vi "Allocate Image Memory.vi"(11 "Reference Image File":string) -> (0 "error out":errorcluster, 1 "Reference Image":T1, 2 "HSL Threshold":T1, 3 "Acquisition Memory":T1[](array[typedef]), 5 "Mask":T1)   [LabVIEW 2018]
uses:
  <vilib>/vision/Image Controls.llb/IMAQ Image.ctl
panel:
  out "appended path":path
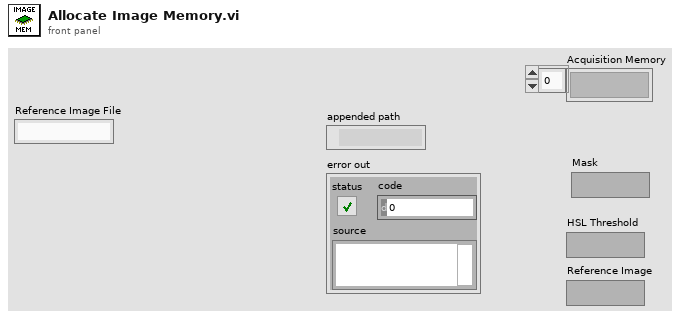
[diagram p1: front panel]
types:
  T1 = typedef "IMAQ Image.ctl" = refnum<image>
  T2 = typedef "Image Type" = u32
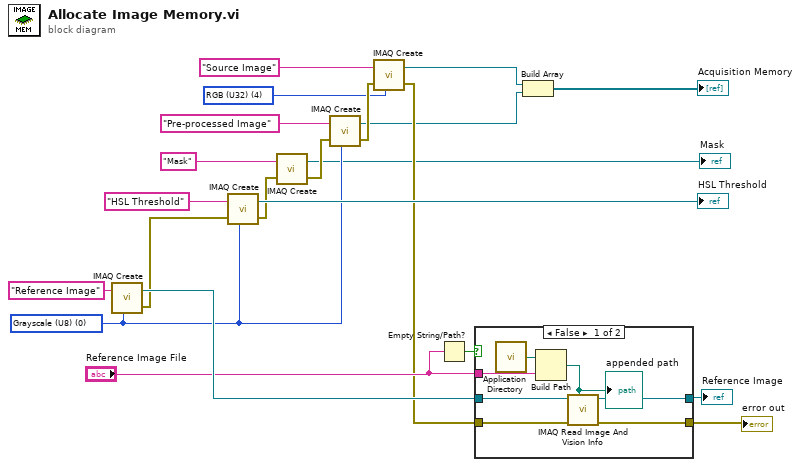
[diagram p0: block diagram]
diagram:
  w7 = T2 4 items=["Grayscale (U8)", "Grayscale (I16)", "Grayscale (SGL)", "Complex (CSG)", "RGB (U32)", "HSL (U32)", "RGB (U64)", "Grayscale (U16)"] ("Image Type")
  w6 = T2 0 items=["Grayscale (U8)", "Grayscale (I16)", "Grayscale (SGL)", "Complex (CSG)", "RGB (U32)", "HSL (U32)", "RGB (U64)", "Grayscale (U16)"] ("Image Type")
  n1 = call "IMAQ Create"("Image Name"="Reference Image", "Image Type"=w6) -> ("New Image"=w22:T1, "error out"=w1:errorcluster)  [unwired: 3 in]
  n2 = call "IMAQ Create"("Image Name"="HSL Threshold", "Image Type"=w6, "error in (no error)"=w1) -> ("New Image"=→"HSL Threshold":T1, "error out"=w5:errorcluster)  [unwired: 2 in]
  n3 = call "IMAQ Create"("Image Name"="Mask", "error in (no error)"=w5) -> ("New Image"=→"Mask":T1, "error out"=w4:errorcluster)  [unwired: 3 in]
  n4 = call "IMAQ Create"("Image Name"="Pre-processed Image", "Image Type"=w6, "error in (no error)"=w4) -> ("New Image"=w10:T1, "error out"=w12:errorcluster)  [unwired: 2 in]
  n5 = call "IMAQ Create"("Image Name"="Source Image", "Image Type"=w7, "error in (no error)"=w12) -> ("New Image"=w9:T1, "error out"=w11:errorcluster)  [unwired: 2 in]
  n6 = Empty String/Path?(string/path="Reference Image File") -> (empty?=w18:bool)
  n7 = case shown="False" w18 {
    tunnel: w22 -> [w27 w31]
    tunnel: "Reference Image File" -> [w26 _]
    tunnel: w11 -> [w25 w30]
    tunnel: [w24 w31] -> w15
    tunnel: [w23 w30] -> w14
    frame False {
      n8 = call <vilib>:"Application Directory.vi"() -> ("Application Directory"=w29:path)
      n9 = Build Path(base path=w29, name or relative path=w26) -> (appended path=w28:path)
      "appended path" <- w28
      n10 = call "IMAQ Read Image And Vision Info"("File Path"=w28, "error in (no error)"=w25, "Image"=w27) -> ("error out"=w23:errorcluster, "Image Out"=w24:T1)  [unwired: 6 in, 1 out]
    }
    frame True {
    }
  }
  "Reference Image" <- w15
  "error out" <- w14
  n11 = Build Array(w9, w10) -> (→"Acquisition Memory":T1[])
